vi "2_0_PatchCore_Inference(Image).vi"() -> ()   [LabVIEW 2020]
uses:
  PatchCore_AddOn/API/Controls/NNPC_Init_Custom_NN_CFG.ctl
  <vilib>/Ngene/Deep Learning Toolkit/Toolkit/NN_Data/API/NN_Dims(C,H,W).ctl
  PatchCore_AddOn/API/Controls/Heatmap_Config.ctl
  PatchCore_AddOn/API/Controls/ColorMap.ctl
  PatchCore_AddOn/API/Controls/MinMax.ctl
  PatchCore_AddOn/API/Controls/Feature_Scorer_Params.ctl
  PatchCore_AddOn/API/Controls/Gaussian_Blur.ctl
  PatchCore_AddOn/API/Controls/NNPC_Device.ctl
  <vilib>/Ngene/Deep Learning Toolkit/Toolkit/NN_Network/Controls/NN_Device.ctl
  PatchCore_AddOn/API/Controls/NNPC_Trained_Model_Paths.ctl
  PatchCore_AddOn/API/Controls/NN_Paths.ctl
  PatchCore_AddOn/API/Controls/NNPC_Save_CFG.ctl
  <vilib>/Utility/miscctls.llb/LVMinMaxIncTypeDef.ctl
  subVIs/Dataset_Reader/Controls/ImRead_PreProcessing_Options.ctl
  PatchCore_AddOn/Low_Level/Controls/Normalization_Type.ctl
  PatchCore_AddOn/API/NNPC_Predict/NNPC_Predict(Single).vi
  PatchCore_AddOn/PatchCore_AddOn.lvlib
  <vilib>/ptbypt/NI_PtbyPt.lvlib
  <vilib>/Ngene/Deep Learning Toolkit/Toolkit/Deep_Learning_Toolkit_by_Ngene.lvlib
panel:
  in  "Cluster":T1
  in  "Trained_Model_Paths":T2={"NNFE_Paths"={"CFG"=path "D:/PatchCore/__24_12_11__22_07_40/wrn_50_2_timm_NNFE__24_12_11__22_07_40.cfg", "BIN"=path "D:/PatchCore/__24_12_11__22_07_40/wrn_50_2_timm_NNFE__24_12_11__22_07_40.bin"}, "PatchCore_Paths"={"CFG"=path "D:/PatchCore/__24_12_11__22_07_40/wrn_50_2_timm_Patchcore__24_12_11__22_07_40.cfg", "BIN"=path "D:/PatchCore/__24_12_11__22_07_40/wrn_50_2_timm_MemBank__PS3_RP296_SR0.1_Size16.4k__24_12_11__22_07_40.bin"}}
  in  "Device_Config.":T4={"Device"=enum."GPU", "GPU Id"=0}
  out "Image_Thrshld (Eval)":sgl=30.7657
  in  "Image_Thrshld(Custom)":sgl=-1.0 format="%_5g"
  out "dT_Predict":dbl=0.010452587000036146 format="%#_3ps"
  out "Pixel_Score(Min)":sgl=1.5847735
  out "Pixel_Score(Max)":sgl=66.74123
  out "Image_File_Path":path=path "D:/MVTec/bottle/test/contamination/018.png"
  in  "Feature_Scorer_Params":T6={"Nearest_Neihbours"=1, "Calculate Anomaly Map"=TRUE, "Gaussian_Blur"={"Kernel_Size"=33, "sigma"=1.0}}
  out "Pixel_Thrshld (Eval)":sgl=25.5661
  in  "Report_Image_Dims":cluster{"X Resolution":i32, "Y Resolution":i32}={"X Resolution"=224, "Y Resolution"=224}
  in  "Stop":bool
  in  "Heatmap_Config":T8={"ColorMap_Type"=enum."Jet", "Alpha"=0.4, "Heatmap Range"={"Min"=-1.0, "Max"=-1.0}} {"Heatmap Range"."Min" format="%#_5g"}
  out "Anomaly?":bool=TRUE
  in  "Eval_Stats_File_Path":path=path "D:/PatchCore/__24_12_11__22_07_40/PatchCore_Eval_Stats__24_12_11__22_13_40.cfg"
  out "dT_ImRead":dbl=0.02295880000019679 format="%#_4ps"
  in  "NNFE_Custom_CFG":T11={"Input3D_Custom_Dims"={"C"=-1, "H"=-1, "W"=-1}, "mBatch"=1}
  out "Anomaly Detection Results":T13(plugin-control)
  out "Img_Score":sgl=67.94195
  in  "Image_idx":u32=80 max=82
  in  "Ground_Truth_Folder_Path":path=path "D:/MVTec/bottle/ground_truth"
  in  "Pixel_Thrshld(Custom)":sgl=-1.0 format="%_5g"
  in  "Test_Dataset_Folder_Path":path=path "D:/MVTec/bottle/test"
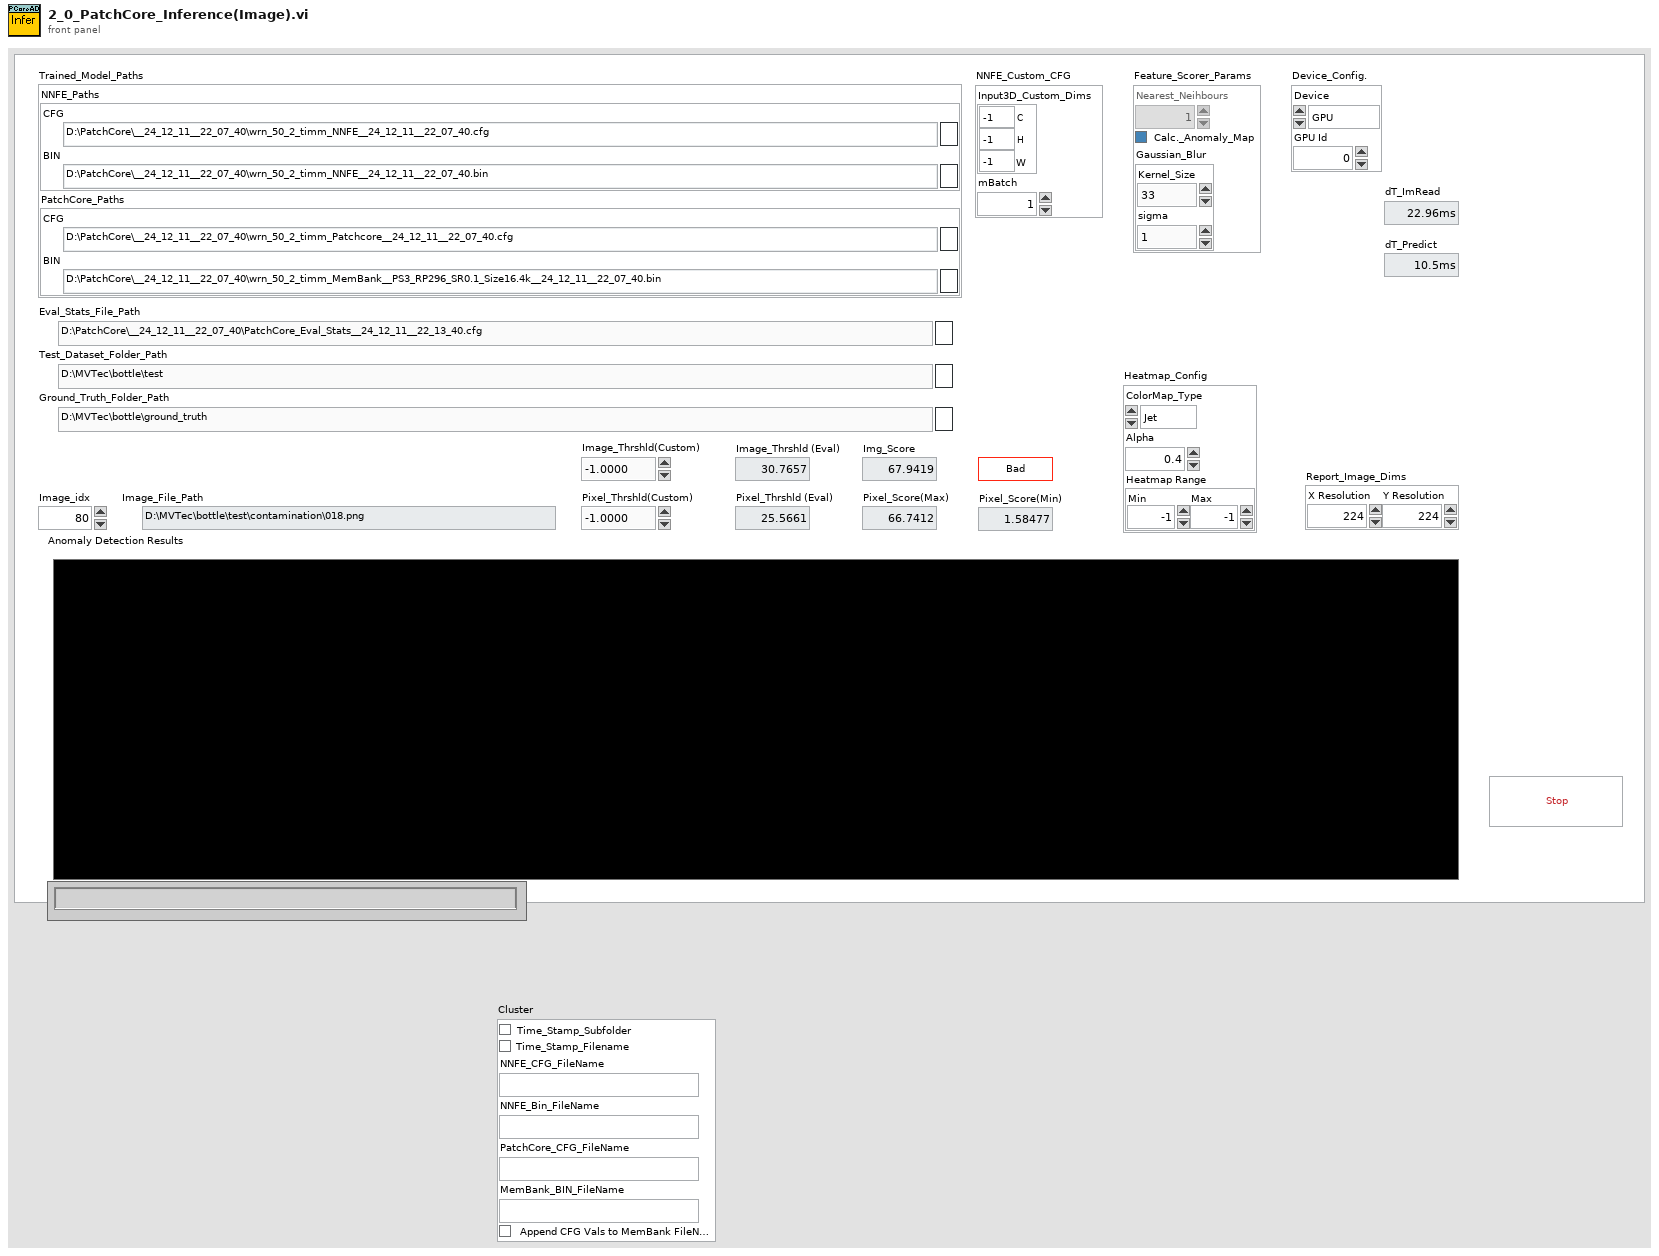
[diagram p1: front panel]
types:
  T1 = typedef "PatchCore_AddOn.lvlib/NNPC_Save_CFG.ctl" = cluster{"Add_TimeStamp_SubFolder":bool, "Append_TimeStamp_to_FileNames":bool, "NNFE_CFG_FileName":string, "NNFE_Bin_FileName":string, "PatchCore_CFG_FileName":string, "MemBank_BIN_FileName":string, "Append_CFG_to_MemBank_FileName":bool}
  T2 = typedef "PatchCore_AddOn.lvlib/NNPC_Trained_Model_Paths.ctl" = cluster{"NNFE_Paths":T3, "PatchCore_Paths":T3}
  T3 = typedef "PatchCore_AddOn.lvlib/NN_Paths.ctl" = cluster{"CFG":path, "BIN":path}
  T4 = typedef "PatchCore_AddOn.lvlib/NNPC_Device.ctl" = cluster{"Device":T5, "GPU Id":i32}
  T5 = typedef "Deep_Learning_Toolkit_by_Ngene.lvlib/NN_Device.ctl" = enum16{"CPU", "GPU"}
  T6 = typedef "PatchCore_AddOn.lvlib/Feature_Scorer_Params.ctl" = cluster{"Nearest_Neihbours":i32, "Calculate Anomaly Map":bool, "Gaussian_Blur":T7}
  T7 = typedef "PatchCore_AddOn.lvlib/Gaussian_Blur.ctl" = cluster{"Kernel_Size":i32, "sigma":sgl}
  T8 = typedef "PatchCore_AddOn.lvlib/Heatmap_Config.ctl" = cluster{"ColorMap_Type":T9, "Alpha":sgl, "Heatmap Range":T10}
  T9 = typedef "PatchCore_AddOn.lvlib/ColorMap.ctl" = enum16{"Jet", "Perula", "Inferno", "Plasma", "Viridis"}
  T10 = typedef "PatchCore_AddOn.lvlib/MinMax.ctl" = cluster{"Min":sgl, "Max":sgl}
  T11 = typedef "PatchCore_AddOn.lvlib/NNPC_Init_Custom_NN_CFG.ctl" = cluster{"Input3D_Custom_Dims":T12, "mBatch":i32}
  T12 = typedef "Deep_Learning_Toolkit_by_Ngene.lvlib/NN_Dims(C,H,W).ctl" = cluster{"C":i32, "H":i32, "W":i32}
  T13 = typedef "IMAQ Image.ctl" = refnum<image>
  T14 = typedef "LVMinMaxIncTypeDef.ctl" = cluster{"Minimum":dbl, "Maximum":dbl, "Increment":dbl}
  T15 = typedef "PatchCore_AddOn.lvlib/NNPC_Instance.ctl" = cluster{"Dataset_Stats":T16, "NN":T18, "Device_Config.":T4, "PatchCore_Init_CFG":T33, "Coreset Params":T35, "MemBank_Data":T37}
  T16 = typedef "PatchCore_AddOn.lvlib/NNPC_DS_Stats.ctl" = cluster{"means":T17, "vars":T17, "DS_Size":i32}
  T17 = typedef "PatchCore_AddOn.lvlib/Image_Stats_RGB.ctl" = cluster{"R":sgl, "G":sgl, "B":sgl}
  T18 = typedef "Deep_Learning_Toolkit_by_Ngene.lvlib/NN.ctl" = cluster{"Name":string, "No of Layers":i32, "mBatch":i32, "Layers":T19[], "Dimty":T20, "Dims_In":T12, "Dims_Out":T12, "Working_Dir":path, "Train?":bool, "Train_Params":T21, "LR_Update_Policy":T24, "Session Data":T26, "Ground_truth":T27, "NNg_hdls":T28, "NN_Device":T5, "GPU Id":i32, "Labels":string[], "Receptive Field":T29[], "Loss_Type":T30, "Loss_Cfg_Prms":variant, "NNG_WS":T31}
  T19 = typedef "Deep_Learning_Toolkit_by_Ngene.lvlib/NN_Layer_ref.ctl" = refnum<data-value>
  T20 = typedef "Deep_Learning_Toolkit_by_Ngene.lvlib/NN_In_Out_Dim-ty.ctl" = enum8{"In1D_Out1D", "In3D_Out1D", "In3D_Out3D", "In3D_OutBBox"}
  T21 = typedef "Deep_Learning_Toolkit_by_Ngene.lvlib/NN_Train_Params.ctl" = cluster{"Optimizer":T22, "Beta_1":sgl, "Beta_2":sgl, "Weight Decay(L1)":sgl, "Weight Decay(L2)":sgl, "Data_Sampling":T23}
  T22 = typedef "Deep_Learning_Toolkit_by_Ngene.lvlib/NN_Train_Optimizer.ctl" = enum16{"SGD", "Adam", "Adagrad", "Adadelta", "RMSProp", "Nesterov"}
  T23 = typedef "Deep_Learning_Toolkit_by_Ngene.lvlib/NN_Train_Data_Sampling.ctl" = enum16{"Random", "Sequential"}
  T24 = typedef "Deep_Learning_Toolkit_by_Ngene.lvlib/NN_LR_Policy_Cfg.ctl" = cluster{"Policy_Type":T25, "LR0":dbl, "k":sgl, "WarmUp_Policy":enum16{"Step", "Ramp"}, "WarmUp_Iter":i32, "WarmUp_Ratio":sgl}
  T25 = typedef "Deep_Learning_Toolkit_by_Ngene.lvlib/NN_LR_Policy_Type.ctl" = enum16{"Manual", "Step", "Exp", "1/t"}
  T26 = typedef "Deep_Learning_Toolkit_by_Ngene.lvlib/NN_Train_Session_Data.ctl" = cluster{"Epochs":sgl, "Tot_Iter":i32, "LR":sgl, "LR_iter":i32}
  T27 = typedef "Deep_Learning_Toolkit_by_Ngene.lvlib/NN_Ground_truth.ctl" = cluster{"Y":variant}
  T28 = typedef "Deep_Learning_Toolkit_by_Ngene.lvlib/nng_cuda_handles.ctl" = cluster{"cudnn":u64, "cublas":u64, "stream":u64, "curand":u64}
  T29 = typedef "Deep_Learning_Toolkit_by_Ngene.lvlib/NN_Dims(V,H).ctl" = cluster{"V":i32, "H":i32}
  T30 = typedef "Deep_Learning_Toolkit_by_Ngene.lvlib/NN_Loss_Type.ctl" = enum16{"None", "MSE", "CrossEntropy", "YOLO_v2", "YOLO_v4"}
  T31 = typedef "Deep_Learning_Toolkit_by_Ngene.lvlib/NNG_WS.ctl" = cluster{"NNG_WS_Mem":T32, "Max_WS_Size":i64}
  T32 = typedef "Deep_Learning_Toolkit_by_Ngene.lvlib/NNg_WS_Mem_DVR.ctl" = refnum<data-value>
  T33 = typedef "PatchCore_AddOn.lvlib/NNPC_Init_CFG.ctl" = cluster{"BackBone":T34, "Out_Layers_Names":string[], "Patch_Size":u32}
  T34 = typedef "PatchCore_AddOn.lvlib/NNPC_BackBone_Selector.ctl" = enum16{"WRN_50_2_L2L3"}
  T35 = typedef "PatchCore_AddOn.lvlib/NNPC_Coreset_Params.ctl" = cluster{"Name":string, "Sampling_Ratio":sgl, "Startd_idx":i32, "Random_Proj?":bool, "Rnd. Proj. Params":T36}
  T36 = typedef "PatchCore_AddOn.lvlib/NNPC_Random_Projection_CFG.ctl" = cluster{"Proj._Dim.":i32, "Epsilon":sgl, "Seed":i32}
  T37 = typedef "PatchCore_AddOn.lvlib/MemBank_and_Norm_Variants.ctl" = cluster{"MemBank":variant, "MemBank Norm":variant}
  T38 = typedef "PatchCore_AddOn.lvlib/Eval_Results.ctl" = cluster{"Scores(Good)":T10, "Scores(Bad)":T10, "F1_Max":sgl, "Thrshld(F1_Max)":sgl, "IoU_Max":sgl, "Thrshld(IoU_Max)":sgl, "AUROC":sgl, "Prec.(F1_Max)":sgl, "Recall(F1_Max)":sgl, "FPR(F1_Max)":sgl, "FNR(F1_Max)":sgl}
  T39 = typedef "ImRead_PreProcessing_Options.ctl" = cluster{"Image Type":T40, "Normalization Type":T41, "Interpolation Type":u32}
  T40 = typedef "Image Type" = u32
  T41 = typedef "PatchCore_AddOn.lvlib/Normalization_Type.ctl" = enum16{"Standardize(DS_Stats)", "Standardize(Image_Stats)"}
  T42 = typedef "PatchCore_AddOn.lvlib/Anomaly_Detection_Results_Imgs.ctl" = cluster{"Image":T13, "Ground Truth":T13, "Predicted Heat Map":T13, "Predicted Mask":T13, "Segmentation":T13}
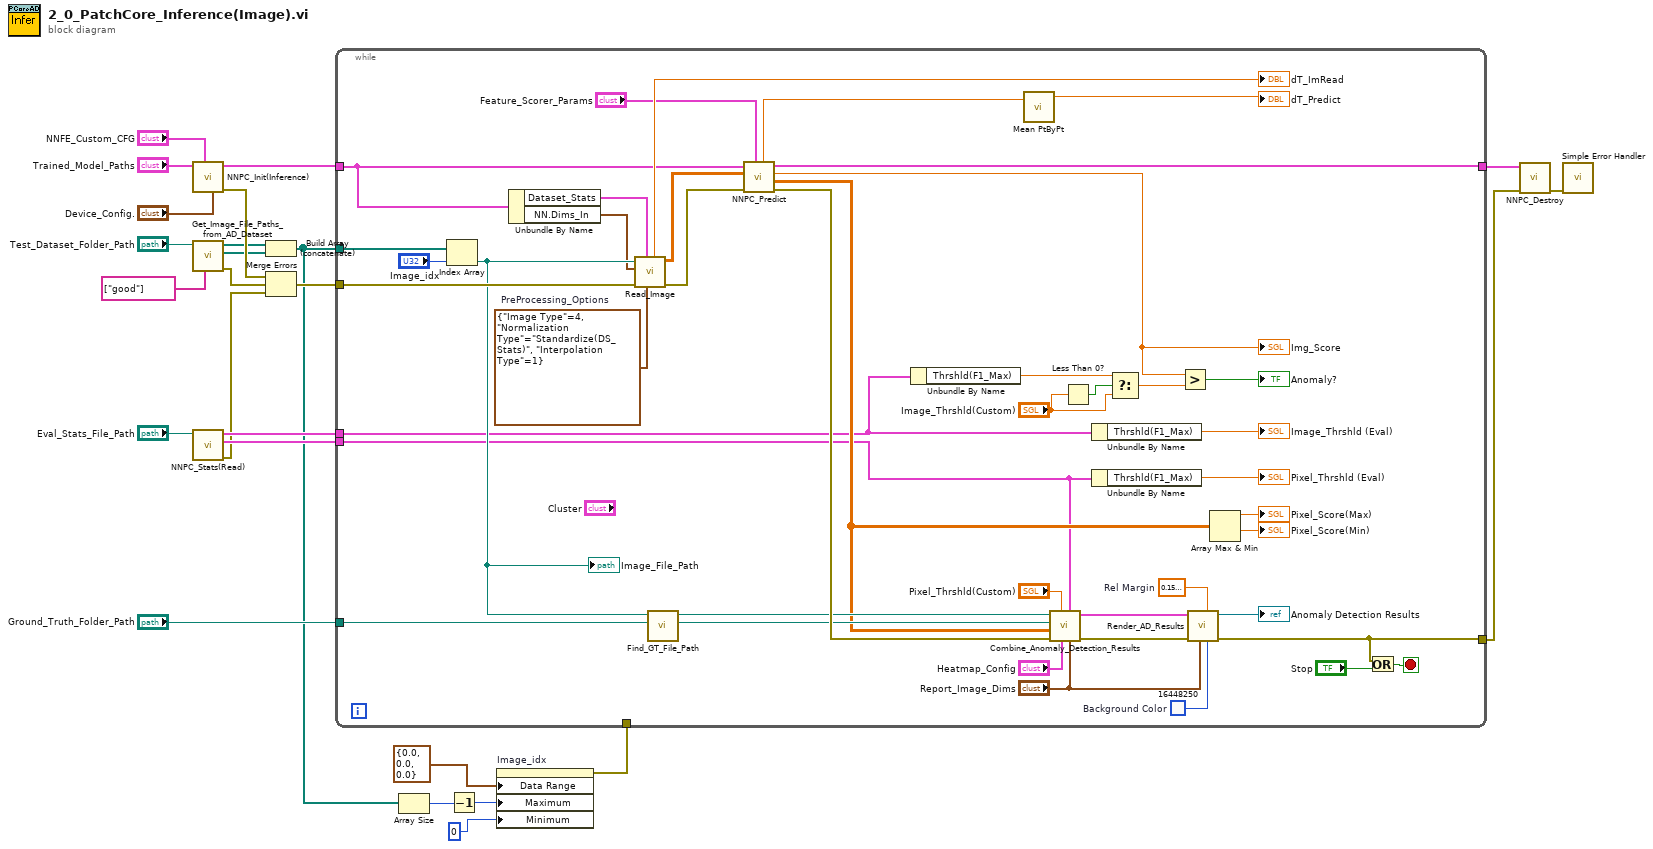
[diagram p0: block diagram]
diagram:
  n1 = call "NNPC_Init(Inference).vi"("Device_Config."="Device_Config.", "NNFE_Custom_CFG"="NNFE_Custom_CFG", "NNFE PatchCore Paths"="Trained_Model_Paths") -> ("error out"=w15:errorcluster, "PCore_Instance out"=w20:T15)  [unwired: 7 in]
  n2 = call "Get_Image_File_Paths_from_AD_Dataset.vi"("Good Folder Names"=string[] ["good"] ("Good Folder Name"), "Dataset Folder"="Test_Dataset_Folder_Path") -> ("error out"=w10:errorcluster, "Bad Dataset Files"=w6:path[], "Good Dataset Files"=w5:path[])  [unwired: 7 in]
  n3 = call "NNPC_Stats(Read).vi"("CFG file path"="Eval_Stats_File_Path") -> ("error out"=w14:errorcluster, "Pixel Results"=w16:T38, "Image Results"=w17:T38)  [unwired: 8 in]
  n4 = Build Array (concatenate)(w5, w6) -> (w11:path[])
  n5 = Merge Errors(w15, w10, w14) -> (w18:errorcluster)
  n6 = Array Size(array=w11) -> (size(s)=w25:i32)
  n7 = Decrement(x=w25) -> (x-1=w24:i32)
  n8 = property on="Image_idx" class="DigNum (strict)"("Data Range"=T14 {"Minimum"=0.0, "Maximum"=0.0, "Increment"=0.0} ("Data Entry Limits"), "Maximum"=w24, "Minimum"=u32 0 ("Data Entry Limits:Minimum")) -> (error out=w4:errorcluster)  [unwired: 2 in, 1 out]
  n9 = while {
    tunnel: w11 -> [w68]
    tunnel: w20 -> [w46]
    tunnel: [w32] -> w8
    tunnel: w17 -> [w39]
    tunnel: w16 -> [w38]
    tunnel: w18 -> [w67]
    tunnel: [w27] -> w9
    tunnel: "Ground_Truth_Folder_Path" -> [w49]
    tunnel: w4 -> [_]
    stop <- w28 stop-if-true
    w26 = u32 16448250  # Background Color
    w59 = sgl 0.15  # Rel Margin
    w33 = T39 {"Image Type"=4, "Normalization Type"=enum."Standardize(DS_Stats)", "Interpolation Type"=1}  # PreProcessing_Options
    n10 = Index Array(array=w68, index="Image_idx") -> (element=w52:path)
    "Image_File_Path" <- w52
    n11 = Unbundle By Name(w46) -> ("Dataset_Stats"=w35:T16, "NN.Dims_In"=w34:T12)
    n12 = call "Read_Image.vi"("PreProcessing_Options"=w33, "Dataset_Stats"=w35, "error in"=w67, "Target_Dims"=w34, "Img Path"=w52) -> ("error out"=w36:errorcluster, "Image Out"=w31:sgl[][][], "dT_Img_Read"=→"dT_ImRead":dbl)  [unwired: 4 in]
    n13 = call "Find_GT_File_Path.vi"("GT Mask Folder Path"=w49, "Image File Path"=w52) -> ("GT File Path"=w50:path, "Image File Path out"=w51:path)  [unwired: 8 in]
    n14 = call-poly "NNPC_Predict.vi"("Feature Scorer Params"="Feature_Scorer_Params", "error in"=w36, "Image in"=w31, "PCore_Instance in"=w46) -> ("error out"=w65:errorcluster, "anomaly map"=w45:sgl[][], "pred score"=w44:sgl, "PCore_Instance out"=w32:T15, "dT_Predict"=w30:dbl)  [unwired: 3 in]
    "Img_Score" <- w44
    n15 = Unbundle By Name(w39) -> ("Thrshld(F1_Max)"=w55:sgl)
    n16 = call <vilib>:"Mean PtByPt.vi"("x"=w30) -> ("mean"=→"dT_Predict":dbl)  [unwired: 3 in, 1 out]
    n17 = call "Combine_Anomaly_Detection_Results.vi"("Infrnc Dims"="Report_Image_Dims", "Pixel Results"=w38, "Heatmap Config"="Heatmap_Config", "Pixel Anomaly Thrshld"="Pixel_Thrshld(Custom)", "error in"=w65, "Anomaly Map"=w45, "Gt File Path"=w50, "Img File Path"=w51) -> ("error out"=w64:errorcluster, "Anomaly Detection Rresults"=w63:T42)  [unwired: 1 in, 1 out]
    n18 = Less Than 0?(x="Image_Thrshld(Custom)") -> (x < 0?=w57:bool)
    n19 = Unbundle By Name(w39) -> ("Thrshld(F1_Max)"=→"Image_Thrshld (Eval)":sgl)
    n20 = Unbundle By Name(w38) -> ("Thrshld(F1_Max)"=→"Pixel_Thrshld (Eval)":sgl)
    n21 = Select(t=w55, s=w57, f="Image_Thrshld(Custom)") -> (s? t:f=w54:sgl)
    n22 = Greater?(x=w44, y=w54) -> (0:→"Anomaly?":bool)
    n23 = call "Render_AD_Results.vi"("Background Color"=w26, "Rel._Margin"=w59, "Image_Dims"="Report_Image_Dims", "error in"=w64, "Anomaly Detection Rresults"=w63) -> ("error out"=w27:errorcluster, "Anomaly Detection Results"=→"Anomaly Detection Results":T13)  [unwired: 5 in]
    n24 = Array Max & Min(array=w45) -> (max value=→"Pixel_Score(Max)":sgl, min value=→"Pixel_Score(Min)":sgl)  [unwired: 2 out]
    n25 = Or(x=w27, y="Stop") -> (x .or. y?=w28:bool)
  }
  n26 = call "NNPC_Destroy.vi"("error in"=w9, "PCore_Instance in"=w8) -> ("error out"=w7:errorcluster)  [unwired: 9 in]
  n27 = call <vilib>:"Simple Error Handler.vi"("error in (no error)"=w7) -> ()  [unwired: 4 in, 5 out]
